vi "ME103 Lab1C SP26.vi"() -> ()   [LabVIEW 2025]
panel:
  out "Voltage Measurements":dynamicdata(graph)
  # "Part 3 - Ping Pong Tower Experimentation"
  # "Use this LabVIEW VI to monitor the voltage output from the IR sensor, and the voltage draw from the fan. Use for hysteresis."
  # "ME 103 Experimentation and Measurements"
  # "Lab 1 Part 3: Ping Pong Tower Experimentation Hysteresis"
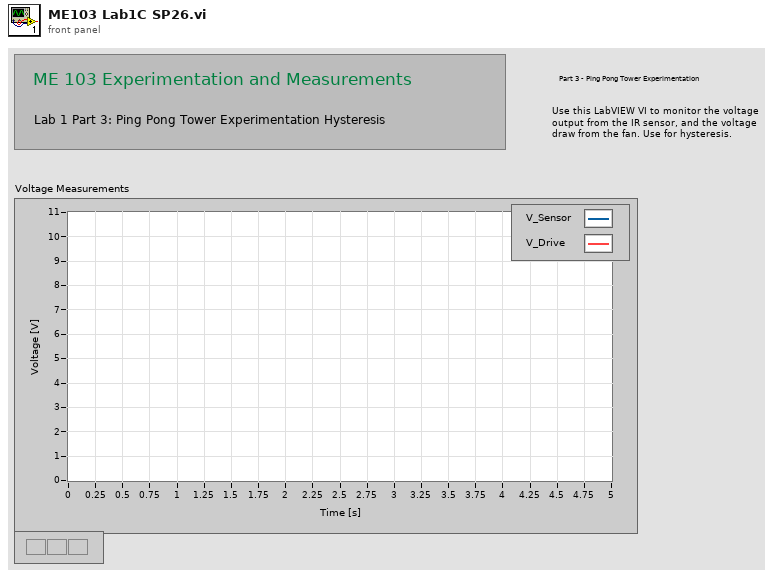
[diagram p1: front panel]
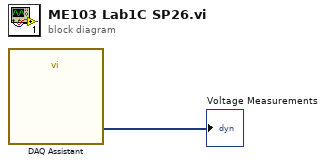
[diagram p0: block diagram]
diagram:
  n1 = call "DAQ Assistant"() -> ("data"=→"Voltage Measurements":dynamicdata)  [unwired: 17 in, 2 out]
